vi "DDS_Clock.vi"() -> ()   [LabVIEW 2016] (continued)
[Hz] CH0"=318400000.0}, {"total time[ms]"=15.450000000000085, "f1 [Hz] CH0"=318200000.0}, {"total time[ms]"=15.450000000000085, "f1 [Hz] CH0"=318200000.0}, {"total time[ms]"=15.500000000000085, "f1 [Hz] CH0"=318000000.0}, {"total time[ms]"=15.500000000000085, "f1 [Hz] CH0"=318000000.0}, {"total time[ms]"=15.550000000000086, "f1 [Hz] CH0"=317800000.0}, {"total time[ms]"=15.550000000000086, "f1 [Hz] CH0"=317800000.0}, {"total time[ms]"=15.600000000000087, "f1 [Hz] CH0"=317600000.0}, {"total time[ms]"=15.600000000000087, "f1 [Hz] CH0"=317600000.0}, {"total time[ms]"=15.650000000000087, "f1 [Hz] CH0"=317400000.0}, {"total time[ms]"=15.650000000000087, "f1 [Hz] CH0"=317400000.0}, {"total time[ms]"=15.700000000000088, "f1 [Hz] CH0"=317200000.0}, {"total time[ms]"=15.700000000000088, "f1 [Hz] CH0"=317200000.0}, {"total time[ms]"=15.750000000000089, "f1 [Hz] CH0"=317000000.0}, {"total time[ms]"=15.750000000000089, "f1 [Hz] CH0"=317000000.0}, {"total time[ms]"=15.80000000000009, "f1 [Hz] CH0"=316800000.0}, {"total time[ms]"=15.80000000000009, "f1 [Hz] CH0"=316800000.0}, {"total time[ms]"=15.85000000000009, "f1 [Hz] CH0"=316600000.0}, {"total time[ms]"=15.85000000000009, "f1 [Hz] CH0"=316600000.0}, {"total time[ms]"=15.900000000000091, "f1 [Hz] CH0"=316400000.0}, {"total time[ms]"=15.900000000000091, "f1 [Hz] CH0"=316400000.0}, {"total time[ms]"=15.950000000000092, "f1 [Hz] CH0"=316200000.0}, {"total time[ms]"=15.950000000000092, "f1 [Hz] CH0"=316200000.0}, {"total time[ms]"=16.000000000000092, "f1 [Hz] CH0"=316000000.0}, {"total time[ms]"=16.000000000000092, "f1 [Hz] CH0"=316000000.0}, {"total time[ms]"=16.050000000000093, "f1 [Hz] CH0"=315800000.0}, {"total time[ms]"=16.050000000000093, "f1 [Hz] CH0"=315800000.0}, {"total time[ms]"=16.100000000000094, "f1 [Hz] CH0"=315600000.0}, {"total time[ms]"=16.100000000000094, "f1 [Hz] CH0"=315600000.0}, {"total time[ms]"=16.150000000000095, "f1 [Hz] CH0"=315400000.0}, {"total time[ms]"=16.150000000000095, "f1 [Hz] CH0"=315400000.0}, {"total time[ms]"=16.200000000000095, "f1 [Hz] CH0"=315200000.0}, {"total time[ms]"=16.200000000000095, "f1 [Hz] CH0"=315200000.0}, {"total time[ms]"=16.250000000000096, "f1 [Hz] CH0"=315000000.0}, {"total time[ms]"=16.250000000000096, "f1 [Hz] CH0"=315000000.0}, {"total time[ms]"=16.300000000000097, "f1 [Hz] CH0"=314800000.0}, {"total time[ms]"=16.300000000000097, "f1 [Hz] CH0"=314800000.0}, {"total time[ms]"=16.350000000000097, "f1 [Hz] CH0"=314600000.0}, {"total time[ms]"=16.350000000000097, "f1 [Hz] CH0"=314600000.0}, {"total time[ms]"=16.400000000000098, "f1 [Hz] CH0"=314400000.0}, {"total time[ms]"=16.400000000000098, "f1 [Hz] CH0"=314400000.0}, {"total time[ms]"=16.4500000000001, "f1 [Hz] CH0"=314200000.0}, {"total time[ms]"=16.4500000000001, "f1 [Hz] CH0"=314200000.0}, {"total time[ms]"=16.5000000000001, "f1 [Hz] CH0"=314000000.0}, {"total time[ms]"=16.5000000000001, "f1 [Hz] CH0"=314000000.0}, {"total time[ms]"=16.5500000000001, "f1 [Hz] CH0"=313800000.0}, {"total time[ms]"=16.5500000000001, "f1 [Hz] CH0"=313800000.0}, {"total time[ms]"=16.6000000000001, "f1 [Hz] CH0"=313600000.0}, {"total time[ms]"=16.6000000000001, "f1 [Hz] CH0"=313600000.0}, {"total time[ms]"=16.6500000000001, "f1 [Hz] CH0"=313400000.0}, {"total time[ms]"=16.6500000000001, "f1 [Hz] CH0"=313400000.0}, {"total time[ms]"=16.700000000000102, "f1 [Hz] CH0"=313200000.0}, {"total time[ms]"=16.700000000000102, "f1 [Hz] CH0"=313200000.0}, {"total time[ms]"=16.750000000000103, "f1 [Hz] CH0"=313000000.0}, {"total time[ms]"=16.750000000000103, "f1 [Hz] CH0"=313000000.0}, {"total time[ms]"=16.800000000000104, "f1 [Hz] CH0"=312800000.0}, {"total time[ms]"=16.800000000000104, "f1 [Hz] CH0"=312800000.0}, {"total time[ms]"=16.850000000000104, "f1 [Hz] CH0"=312600000.0}, {"total time[ms]"=16.850000000000104, "f1 [Hz] CH0"=312600000.0}, {"total time[ms]"=16.900000000000105, "f1 [Hz] CH0"=312400000.0}, {"total time[ms]"=16.900000000000105, "f1 [Hz] CH0"=312400000.0}, {"total time[ms]"=16.950000000000106, "f1 [Hz] CH0"=312200000.0}, {"total time[ms]"=16.950000000000106, "f1 [Hz] CH0"=312200000.0}, {"total time[ms]"=17.000000000000107, "f1 [Hz] CH0"=312000000.0}, {"total time[ms]"=17.000000000000107, "f1 [Hz] CH0"=312000000.0}, {"total time[ms]"=17.050000000000107, "f1 [Hz] CH0"=311800000.0}, {"total time[ms]"=17.050000000000107, "f1 [Hz] CH0"=311800000.0}, {"total time[ms]"=17.100000000000108, "f1 [Hz] CH0"=311600000.0}, {"total time[ms]"=17.100000000000108, "f1 [Hz] CH0"=311600000.0}, {"total time[ms]"=17.15000000000011, "f1 [Hz] CH0"=311400000.0}, {"total time[ms]"=17.15000000000011, "f1 [Hz] CH0"=311400000.0}, {"total time[ms]"=17.20000000000011, "f1 [Hz] CH0"=311200000.0}, {"total time[ms]"=17.20000000000011, "f1 [Hz] CH0"=311200000.0}, {"total time[ms]"=17.25000000000011, "f1 [Hz] CH0"=311000000.0}, {"total time[ms]"=17.25000000000011, "f1 [Hz] CH0"=311000000.0}, {"total time[ms]"=17.30000000000011, "f1 [Hz] CH0"=310800000.0}, {"total time[ms]"=17.30000000000011, "f1 [Hz] CH0"=310800000.0}, {"total time[ms]"=17.35000000000011, "f1 [Hz] CH0"=310600000.0}, {"total time[ms]"=17.35000000000011, "f1 [Hz] CH0"=310600000.0}, {"total time[ms]"=17.400000000000112, "f1 [Hz] CH0"=310400000.0}, {"total time[ms]"=17.400000000000112, "f1 [Hz] CH0"=310400000.0}, {"total time[ms]"=17.450000000000113, "f1 [Hz] CH0"=310200000.0}, {"total time[ms]"=17.450000000000113, "f1 [Hz] CH0"=310200000.0}, {"total time[ms]"=17.500000000000114, "f1 [Hz] CH0"=310000000.0}, {"total time[ms]"=17.500000000000114, "f1 [Hz] CH0"=310000000.0}, {"total time[ms]"=17.550000000000114, "f1 [Hz] CH0"=309800000.0}, {"total time[ms]"=17.550000000000114, "f1 [Hz] CH0"=309800000.0}, {"total time[ms]"=17.600000000000115, "f1 [Hz] CH0"=309600000.0}, {"total time[ms]"=17.600000000000115, "f1 [Hz] CH0"=309600000.0}, {"total time[ms]"=17.650000000000116, "f1 [Hz] CH0"=309400000.0}, {"total time[ms]"=17.650000000000116, "f1 [Hz] CH0"=309400000.0}, {"total time[ms]"=17.700000000000117, "f1 [Hz] CH0"=309200000.0}, {"total time[ms]"=17.700000000000117, "f1 [Hz] CH0"=309200000.0}, {"total time[ms]"=17.750000000000117, "f1 [Hz] CH0"=309000000.0}, {"total time[ms]"=17.750000000000117, "f1 [Hz] CH0"=309000000.0}, {"total time[ms]"=17.800000000000118, "f1 [Hz] CH0"=308800000.0}, {"total time[ms]"=17.800000000000118, "f1 [Hz] CH0"=308800000.0}, {"total time[ms]"=17.85000000000012, "f1 [Hz] CH0"=308600000.0}, {"total time[ms]"=17.85000000000012, "f1 [Hz] CH0"=308600000.0}, {"total time[ms]"=17.90000000000012, "f1 [Hz] CH0"=308400000.0}, {"total time[ms]"=17.90000000000012, "f1 [Hz] CH0"=308400000.0}, {"total time[ms]"=17.95000000000012, "f1 [Hz] CH0"=308200000.0}, {"total time[ms]"=17.95000000000012, "f1 [Hz] CH0"=308200000.0}, {"total time[ms]"=18.00000000000012, "f1 [Hz] CH0"=308000000.0}, {"total time[ms]"=18.00000000000012, "f1 [Hz] CH0"=308000000.0}, {"total time[ms]"=18.05000000000012, "f1 [Hz] CH0"=307800000.0}, {"total time[ms]"=18.05000000000012, "f1 [Hz] CH0"=307800000.0}, {"total time[ms]"=18.100000000000122, "f1 [Hz] CH0"=307600000.0}, {"total time[ms]"=18.100000000000122, "f1 [Hz] CH0"=307600000.0}, {"total time[ms]"=18.150000000000123, "f1 [Hz] CH0"=307400000.0}, {"total time[ms]"=18.150000000000123, "f1 [Hz] CH0"=307400000.0}, {"total time[ms]"=18.200000000000124, "f1 [Hz] CH0"=307200000.0}, {"total time[ms]"=18.200000000000124, "f1 [Hz] CH0"=307200000.0}, {"total time[ms]"=18.250000000000124, "f1 [Hz] CH0"=307000000.0}, {"total time[ms]"=18.250000000000124, "f1 [Hz] CH0"=307000000.0}, {"total time[ms]"=18.300000000000125, "f1 [Hz] CH0"=306800000.0}, {"total time[ms]"=18.300000000000125, "f1 [Hz] CH0"=306800000.0}, {"total time[ms]"=18.350000000000126, "f1 [Hz] CH0"=306600000.0}, {"total time[ms]"=18.350000000000126, "f1 [Hz] CH0"=306600000.0}, {"total time[ms]"=18.400000000000126, "f1 [Hz] CH0"=306400000.0}, {"total time[ms]"=18.400000000000126, "f1 [Hz] CH0"=306400000.0}, {"total time[ms]"=18.450000000000127, "f1 [Hz] CH0"=306200000.0}, {"total time[ms]"=18.450000000000127, "f1 [Hz] CH0"=306200000.0}, {"total time[ms]"=18.500000000000128, "f1 [Hz] CH0"=306000000.0}, {"total time[ms]"=18.500000000000128, "f1 [Hz] CH0"=306000000.0}, {"total time[ms]"=18.55000000000013, "f1 [Hz] CH0"=305800000.0}, {"total time[ms]"=18.55000000000013, "f1 [Hz] CH0"=305800000.0}, {"total time[ms]"=18.60000000000013, "f1 [Hz] CH0"=305600000.0}, {"total time[ms]"=18.60000000000013, "f1 [Hz] CH0"=305600000.0}, {"total time[ms]"=18.65000000000013, "f1 [Hz] CH0"=305400000.0}, {"total time[ms]"=18.65000000000013, "f1 [Hz] CH0"=305400000.0}, {"total time[ms]"=18.70000000000013, "f1 [Hz] CH0"=305200000.0}, {"total time[ms]"=18.70000000000013, "f1 [Hz] CH0"=305200000.0}, {"total time[ms]"=18.75000000000013, "f1 [Hz] CH0"=305000000.0}, {"total time[ms]"=18.75000000000013, "f1 [Hz] CH0"=305000000.0}, {"total time[ms]"=18.800000000000132, "f1 [Hz] CH0"=304800000.0}, {"total time[ms]"=18.800000000000132, "f1 [Hz] CH0"=304800000.0}, {"total time[ms]"=18.850000000000133, "f1 [Hz] CH0"=304600000.0}, {"total time[ms]"=18.850000000000133, "f1 [Hz] CH0"=304600000.0}, {"total time[ms]"=18.900000000000134, "f1 [Hz] CH0"=304400000.0}, {"total time[ms]"=18.900000000000134, "f1 [Hz] CH0"=304400000.0}, {"total time[ms]"=18.950000000000134, "f1 [Hz] CH0"=304200000.0}, {"total time[ms]"=18.950000000000134, "f1 [Hz] CH0"=304200000.0}, {"total time[ms]"=19.000000000000135, "f1 [Hz] CH0"=304000000.0}, {"total time[ms]"=19.000000000000135, "f1 [Hz] CH0"=304000000.0}, {"total time[ms]"=19.050000000000136, "f1 [Hz] CH0"=303800000.0}, {"total time[ms]"=19.050000000000136, "f1 [Hz] CH0"=303800000.0}, {"total time[ms]"=19.100000000000136, "f1 [Hz] CH0"=303600000.0}, {"total time[ms]"=19.100000000000136, "f1 [Hz] CH0"=303600000.0}, {"total time[ms]"=19.150000000000137, "f1 [Hz] CH0"=303400000.0}, {"total time[ms]"=19.150000000000137, "f1 [Hz] CH0"=303400000.0}, {"total time[ms]"=19.200000000000138, "f1 [Hz] CH0"=303200000.0}, {"total time[ms]"=19.200000000000138, "f1 [Hz] CH0"=303200000.0}, {"total time[ms]"=19.25000000000014, "f1 [Hz] CH0"=303000000.0}, {"total time[ms]"=19.25000000000014, "f1 [Hz] CH0"=303000000.0}, {"total time[ms]"=19.30000000000014, "f1 [Hz] CH0"=302800000.0}, {"total time[ms]"=19.30000000000014, "f1 [Hz] CH0"=302800000.0}, {"total time[ms]"=19.35000000000014, "f1 [Hz] CH0"=302600000.0}, {"total time[ms]"=19.35000000000014, "f1 [Hz] CH0"=302600000.0}, {"total time[ms]"=19.40000000000014, "f1 [Hz] CH0"=302400000.0}, {"total time[ms]"=19.40000000000014, "f1 [Hz] CH0"=302400000.0}, {"total time[ms]"=19.45000000000014, "f1 [Hz] CH0"=302200000.0}, {"total time[ms]"=19.45000000000014, "f1 [Hz] CH0"=302200000.0}, {"total time[ms]"=19.500000000000142, "f1 [Hz] CH0"=302000000.0}, {"total time[ms]"=19.500000000000142, "f1 [Hz] CH0"=302000000.0}, {"total time[ms]"=19.550000000000143, "f1 [Hz] CH0"=301800000.0}, {"total time[ms]"=19.550000000000143, "f1 [Hz] CH0"=301800000.0}, {"total time[ms]"=19.600000000000144, "f1 [Hz] CH0"=301600000.0}, {"total time[ms]"=19.600000000000144, "f1 [Hz] CH0"=301600000.0}, {"total time[ms]"=19.650000000000144, "f1 [Hz] CH0"=301400000.0}, {"total time[ms]"=19.650000000000144, "f1 [Hz] CH0"=301400000.0}, {"total time[ms]"=19.700000000000145, "f1 [Hz] CH0"=301200000.0}, {"total time[ms]"=19.700000000000145, "f1 [Hz] CH0"=301200000.0}, {"total time[ms]"=19.750000000000146, "f1 [Hz] CH0"=301000000.0}, {"total time[ms]"=19.750000000000146, "f1 [Hz] CH0"=301000000.0}, {"total time[ms]"=19.800000000000146, "f1 [Hz] CH0"=300800000.0}, {"total time[ms]"=19.800000000000146, "f1 [Hz] CH0"=300800000.0}, {"total time[ms]"=19.850000000000147, "f1 [Hz] CH0"=300600000.0}, {"total time[ms]"=19.850000000000147, "f1 [Hz] CH0"=300600000.0}, {"total time[ms]"=19.900000000000148, "f1 [Hz] CH0"=300400000.0}, {"total time[ms]"=19.900000000000148, "f1 [Hz] CH0"=300400000.0}, {"total time[ms]"=19.95000000000015, "f1 [Hz] CH0"=300200000.0}, {"total time[ms]"=19.95000000000015, "f1 [Hz] CH0"=300200000.0}, {"total time[ms]"=20.00000000000015, "f1 [Hz] CH0"=300000000.0}, {"total time[ms]"=20.00000000000015, "f1 [Hz] CH0"=300000000.0}, {"total time[ms]"=20.05000000000015, "f1 [Hz] CH0"=300200000.0}, {"total time[ms]"=20.05000000000015, "f1 [Hz] CH0"=300200000.0}, {"total time[ms]"=20.10000000000015, "f1 [Hz] CH0"=300400000.0}, {"total time[ms]"=20.10000000000015, "f1 [Hz] CH0"=300400000.0}, {"total time[ms]"=20.15000000000015, "f1 [Hz] CH0"=300600000.0}, {"total time[ms]"=20.15000000000015, "f1 [Hz] CH0"=300600000.0}, {"total time[ms]"=20.200000000000152, "f1 [Hz] CH0"=300800000.0}, {"total time[ms]"=20.200000000000152, "f1 [Hz] CH0"=300800000.0}, {"total time[ms]"=20.250000000000153, "f1 [Hz] CH0"=301000000.0}, {"total time[ms]"=20.250000000000153, "f1 [Hz] CH0"=301000000.0}, {"total time[ms]"=20.300000000000153, "f1 [Hz] CH0"=301200000.0}, {"total time[ms]"=20.300000000000153, "f1 [Hz] CH0"=301200000.0}, {"total time[ms]"=20.350000000000154, "f1 [Hz] CH0"=301400000.0}, {"total time[ms]"=20.350000000000154, "f1 [Hz] CH0"=301400000.0}, {"total time[ms]"=20.400000000000155, "f1 [Hz] CH0"=301600000.0}, {"total time[ms]"=20.400000000000155, "f1 [Hz] CH0"=301600000.0}, {"total time[ms]"=20.450000000000156, "f1 [Hz] CH0"=301800000.0}, {"total time[ms]"=20.450000000000156, "f1 [Hz] CH0"=301800000.0}, {"total time[ms]"=20.500000000000156, "f1 [Hz] CH0"=302000000.0}, {"total time[ms]"=20.500000000000156, "f1 [Hz] CH0"=302000000.0}, {"total time[ms]"=20.550000000000157, "f1 [Hz] CH0"=302200000.0}, {"total time[ms]"=20.550000000000157, "f1 [Hz] CH0"=302200000.0}, {"total time[ms]"=20.600000000000158, "f1 [Hz] CH0"=302400000.0}, {"total time[ms]"=20.600000000000158, "f1 [Hz] CH0"=302400000.0}, {"total time[ms]"=20.65000000000016, "f1 [Hz] CH0"=302600000.0}, {"total time[ms]"=20.65000000000016, "f1 [Hz] CH0"=302600000.0}, {"total time[ms]"=20.70000000000016, "f1 [Hz] CH0"=302800000.0}, {"total time[ms]"=20.70000000000016, "f1 [Hz] CH0"=302800000.0}, {"total time[ms]"=20.75000000000016, "f1 [Hz] CH0"=303000000.0}, {"total time[ms]"=20.75000000000016, "f1 [Hz] CH0"=303000000.0}, {"total time[ms]"=20.80000000000016, "f1 [Hz] CH0"=303200000.0}, {"total time[ms]"=20.80000000000016, "f1 [Hz] CH0"=303200000.0}, {"total time[ms]"=20.85000000000016, "f1 [Hz] CH0"=303400000.0}, {"total time[ms]"=20.85000000000016, "f1 [Hz] CH0"=303400000.0}, {"total time[ms]"=20.900000000000162, "f1 [Hz] CH0"=303600000.0}, {"total time[ms]"=20.900000000000162, "f1 [Hz] CH0"=303600000.0}, {"total time[ms]"=20.950000000000163, "f1 [Hz] CH0"=303800000.0}, {"total time[ms]"=20.950000000000163, "f1 [Hz] CH0"=303800000.0}, {"total time[ms]"=21.000000000000163, "f1 [Hz] CH0"=304000000.0}, {"total time[ms]"=21.000000000000163, "f1 [Hz] CH0"=304000000.0}, {"total time[ms]"=21.050000000000164, "f1 [Hz] CH0"=304200000.0}, {"total time[ms]"=21.050000000000164, "f1 [Hz] CH0"=304200000.0}, {"total time[ms]"=21.100000000000165, "f1 [Hz] CH0"=304400000.0}, {"total time[ms]"=21.100000000000165, "f1 [Hz] CH0"=304400000.0}, {"total time[ms]"=21.150000000000166, "f1 [Hz] CH0"=304600000.0}, {"total time[ms]"=21.150000000000166, "f1 [Hz] CH0"=304600000.0}, {"total time[ms]"=21.200000000000166, "f1 [Hz] CH0"=304800000.0}, {"total time[ms]"=21.200000000000166, "f1 [Hz] CH0"=304800000.0}, {"total time[ms]"=21.250000000000167, "f1 [Hz] CH0"=305000000.0}, {"total time[ms]"=21.250000000000167, "f1 [Hz] CH0"=305000000.0}, {"total time[ms]"=21.300000000000168, "f1 [Hz] CH0"=305200000.0}, {"total time[ms]"=21.300000000000168, "f1 [Hz] CH0"=305200000.0}, {"total time[ms]"=21.35000000000017, "f1 [Hz] CH0"=305400000.0}, {"total time[ms]"=21.35000000000017, "f1 [Hz] CH0"=305400000.0}, {"total time[ms]"=21.40000000000017, "f1 [Hz] CH0"=305600000.0}, {"total time[ms]"=21.40000000000017, "f1 [Hz] CH0"=305600000.0}, {"total time[ms]"=21.45000000000017, "f1 [Hz] CH0"=305800000.0}, {"total time[ms]"=21.45000000000017, "f1 [Hz] CH0"=305800000.0}, {"total time[ms]"=21.50000000000017, "f1 [Hz] CH0"=306000000.0}, {"total time[ms]"=21.50000000000017, "f1 [Hz] CH0"=306000000.0}, {"total time[ms]"=21.55000000000017, "f1 [Hz] CH0"=306200000.0}, {"total time[ms]"=21.55000000000017, "f1 [Hz] CH0"=306200000.0}, {"total time[ms]"=21.600000000000172, "f1 [Hz] CH0"=306400000.0}, {"total time[ms]"=21.600000000000172, "f1 [Hz] CH0"=306400000.0}, {"total time[ms]"=21.650000000000173, "f1 [Hz] CH0"=306600000.0}, {"total time[ms]"=21.650000000000173, "f1 [Hz] CH0"=306600000.0}, {"total time[ms]"=21.700000000000173, "f1 [Hz] CH0"=306800000.0}, {"total time[ms]"=21.700000000000173, "f1 [Hz] CH0"=306800000.0}, {"total time[ms]"=21.750000000000174, "f1 [Hz] CH0"=307000000.0}, {"total time[ms]"=21.750000000000174, "f1 [Hz] CH0"=307000000.0}, {"total time[ms]"=21.800000000000175, "f1 [Hz] CH0"=307200000.0}, {"total time[ms]"=21.800000000000175, "f1 [Hz] CH0"=307200000.0}, {"total time[ms]"=21.850000000000176, "f1 [Hz] CH0"=307400000.0}, {"total time[ms]"=21.850000000000176, "f1 [Hz] CH0"=307400000.0}, {"total time[ms]"=21.900000000000176, "f1 [Hz] CH0"=307600000.0}, {"total time[ms]"=21.900000000000176, "f1 [Hz] CH0"=307600000.0}, {"total time[ms]"=21.950000000000177, "f1 [Hz] CH0"=307800000.0}, {"total time[ms]"=21.950000000000177, "f1 [Hz] CH0"=307800000.0}, {"total time[ms]"=22.000000000000178, "f1 [Hz] CH0"=308000000.0}, {"total time[ms]"=22.000000000000178, "f1 [Hz] CH0"=308000000.0}, {"total time[ms]"=22.05000000000018, "f1 [Hz] CH0"=308200000.0}, {"total time[ms]"=22.05000000000018, "f1 [Hz] CH0"=308200000.0}, {"total time[ms]"=22.10000000000018, "f1 [Hz] CH0"=308400000.0}, {"total time[ms]"=22.10000000000018, "f1 [Hz] CH0"=308400000.0}, {"total time[ms]"=22.15000000000018, "f1 [Hz] CH0"=308600000.0}, {"total time[ms]"=22.15000000000018, "f1 [Hz] CH0"=308600000.0}, {"total time[ms]"=22.20000000000018, "f1 [Hz] CH0"=308800000.0}, {"total time[ms]"=22.20000000000018, "f1 [Hz] CH0"=308800000.0}, {"total time[ms]"=22.25000000000018, "f1 [Hz] CH0"=309000000.0}, {"total time[ms]"=22.25000000000018, "f1 [Hz] CH0"=309000000.0}, {"total time[ms]"=22.300000000000182, "f1 [Hz] CH0"=309200000.0}, {"total time[ms]"=22.300000000000182, "f1 [Hz] CH0"=309200000.0}, {"total time[ms]"=22.350000000000183, "f1 [Hz] CH0"=309400000.0}, {"total time[ms]"=22.350000000000183, "f1 [Hz] CH0"=309400000.0}, {"total time[ms]"=22.400000000000183, "f1 [Hz] CH0"=309600000.0}, {"total time[ms]"=22.400000000000183, "f1 [Hz] CH0"=309600000.0}, {"total time[ms]"=22.450000000000184, "f1 [Hz] CH0"=309800000.0}, {"total time[ms]"=22.450000000000184, "f1 [Hz] CH0"=309800000.0}, {"total time[ms]"=22.500000000000185, "f1 [Hz] CH0"=310000000.0}, {"total time[ms]"=22.500000000000185, "f1 [Hz] CH0"=310000000.0}, {"total time[ms]"=22.550000000000185, "f1 [Hz] CH0"=310200000.0}, {"total time[ms]"=22.550000000000185, "f1 [Hz] CH0"=310200000.0}, {"total time[ms]"=22.600000000000186, "f1 [Hz] CH0"=310400000.0}, {"total time[ms]"=22.600000000000186, "f1 [Hz] CH0"=310400000.0}, {"total time[ms]"=22.650000000000187, "f1 [Hz] CH0"=310600000.0}, {"total time[ms]"=22.650000000000187, "f1 [Hz] CH0"=310600000.0}, {"total time[ms]"=22.700000000000188, "f1 [Hz] CH0"=310800000.0}, {"total time[ms]"=22.700000000000188, "f1 [Hz] CH0"=310800000.0}, {"total time[ms]"=22.75000000000019, "f1 [Hz] CH0"=311000000.0}, {"total time[ms]"=22.75000000000019, "f1 [Hz] CH0"=311000000.0}, {"total time[ms]"=22.80000000000019, "f1 [Hz] CH0"=311200000.0}, {"total time[ms]"=22.80000000000019, "f1 [Hz] CH0"=311200000.0}, {"total time[ms]"=22.85000000000019, "f1 [Hz] CH0"=311400000.0}, {"total time[ms]"=22.85000000000019, "f1 [Hz] CH0"=311400000.0}, {"total time[ms]"=22.90000000000019, "f1 [Hz] CH0"=311600000.0}, {"total time[ms]"=22.90000000000019, "f1 [Hz] CH0"=311600000.0}, {"total time[ms]"=22.95000000000019, "f1 [Hz] CH0"=311800000.0}, {"total time[ms]"=22.95000000000019, "f1 [Hz] CH0"=311800000.0}, {"total time[ms]"=23.000000000000192, "f1 [Hz] CH0"=312000000.0}, {"total time[ms]"=23.000000000000192, "f1 [Hz] CH0"=312000000.0}, {"total time[ms]"=23.050000000000193, 
